vi "Init.vi"(8 "error in (no error)":errorcluster, 11 "Domain_Steady":refnum<class "NI_Domain_Steady.lvclass">) -> (0 "error out":errorcluster, 3 "initialized Domain_Steady":refnum<class "NI_Domain_Steady.lvclass">)   [LabVIEW 2017, in "NI_PDE.lvlib" / "NI_Domain_Steady.lvclass"]
uses:
  <vilib>/gmath/pde.llb/DomainClass/Domain_Steady/NI_Domain_Steady.lvclass
  <vilib>/gmath/pde.llb/DomainClass/Class Type.ctl
  <vilib>/gmath/pde.llb/DomainClass/NI_Domain.lvclass
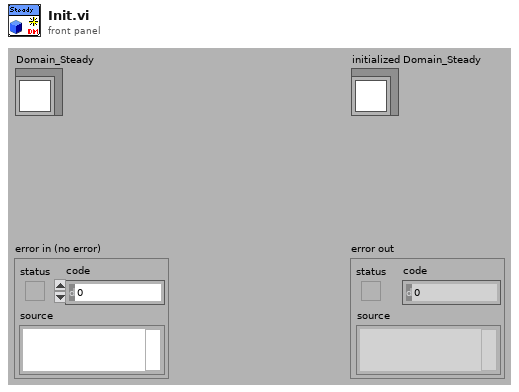
[diagram p1: front panel]
types:
  T1 = typedef "NI_PDE.lvlib/NI_Domain.lvclass/Class Type.ctl" = i32
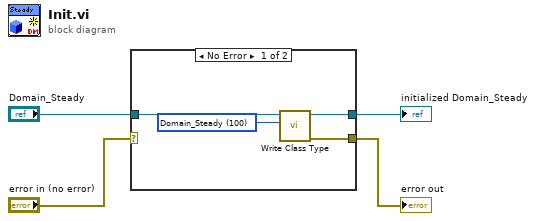
[diagram p0: block diagram]
diagram:
  n1 = case shown="No Error" "error in (no error)" {
    selector: "error in (no error)" -> [_ w10]
    tunnel: "Domain_Steady" -> [w7 w9]
    tunnel: [w6 w10] -> w3
    tunnel: [w5 w9] -> w2
    frame No Error {
      w8 = T1 100 items=["Domain"=0, "Domain_Steady"=100, "Domain_Steady_2D_Rect"=121, "Domain_Steady_2D_Polygon"=122, "Domain_Evolut"=200, "Domain_Evolut_1D"=210, "Domain_Evolut_2D_Rect"=221] ("domain class type")
      n2 = call-dynamic "Write Class Type.vi"("domain class type"=w8, "Domain.lvclass in"=w7) -> ("error out"=w6:errorcluster, "Domain.lvclass out"=w5:refnum<class "NI_Domain_Steady.lvclass">)  [unwired: 1 in, 7 out]
    }
    frame Error {
    }
  }
  "initialized Domain_Steady" <- w2
  "error out" <- w3
